vi "GetFileListing.vi"(10 "patterns":string[](array[string])=["*.py"], 11 "Base Path":path) -> (0 "error out":errorcluster, 1 "Files":path[](array[path]), 2 "All Files":path[](array[path]), 3 "Base":path)   [LabVIEW 2020]
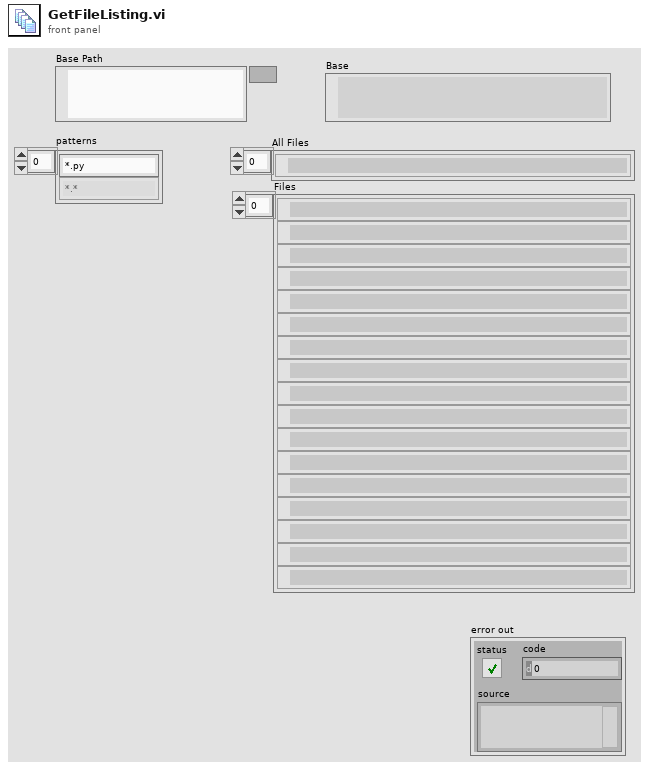
[diagram p1: front panel]
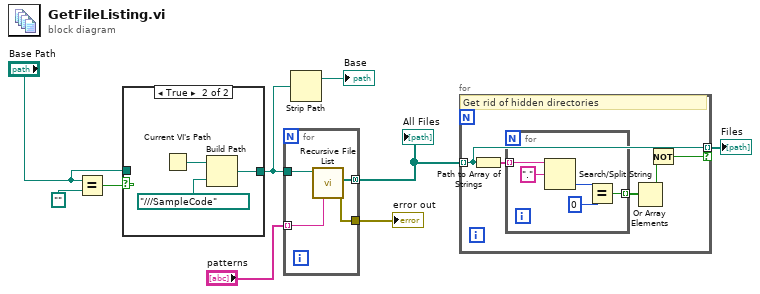
[diagram p0: block diagram]
diagram:
  n1 = Equal?(x="Base Path", y=path "") -> (x = y?=w4:bool)
  n2 = case shown="True" w4 {
    tunnel: [w10 w11] -> w7
    tunnel: "Base Path" -> [w10 _]
    frame False {
    }
    frame True {
      n3 = Current VI's Path() -> (path=w13:path)
      n4 = Build Path(base path=w13, name or relative path=path "../../../SampleCode") -> (appended path=w11:path)
    }
  }
  n5 = for {
    tunnel: [w17] -> w1 mode=concatenating
    tunnel: [w16] -> w2
    tunnel: "patterns" -> [w15] mode=indexing
    tunnel: w7 -> [w14]
    n6 = call <vilib>:"Recursive File List.vi"("pattern"=w15, "Folder Path"=w14) -> ("error out"=w16:errorcluster, "All Files in Dir"=w17:path[])  [unwired: 5 in, 3 out]
  }
  "All Files" <- w1
  "error out" <- w2
  n7 = Strip Path(path=w7) -> (stripped path=→"Base":path)  [unwired: 1 out]
  n8 = for {
    tunnel: w1 -> [w20] mode=indexing
    tunnel: [w20] -> w8 mode=indexing if=w18
    # "Get rid of hidden directories"
    n9 = Path to Array of Strings(0:w20) -> (2:w22:string[])  [unwired: 1 out]
    n10 = for {
      tunnel: w22 -> [w27] mode=indexing
      tunnel: [w23] -> w21 mode=indexing
      n11 = Search/Split String(string=w27, search string/char (-)=".") -> (offset of match=w25:i32)  [unwired: 1 in, 2 out]
      n12 = Equal?(x=w25, y=0) -> (x = y?=w23:bool)
    }
    n13 = Or Array Elements(Boolean array=w21) -> (logical OR=w19:bool)
    n14 = Not(x=w19) -> (.not. x?=w18:bool)
  }
  "Files" <- w8
